vi "Update DropdownMenu.vi"(10 "VacuumLine Obj":refnum<class "VacuumLine.lvclass">, 11 "Controls[]":refnum<vi>[](array[refnum])) -> ()   [LabVIEW 2016, in "Hardware.lvlib" / "VacuumLine.lvlib" / "VacuumLine Configuration.lvclass"]
uses:
  <userlib>/Common Components/Hardware/Abstract System/VacuumLine/VacuumLine Config/VacuumLine Configuration.lvclass
  <userlib>/Common Components/Hardware/Abstract System/VacuumLine/VacuumLine/VacuumLine.lvclass
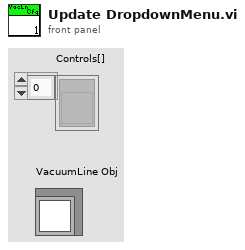
[diagram p1: front panel]
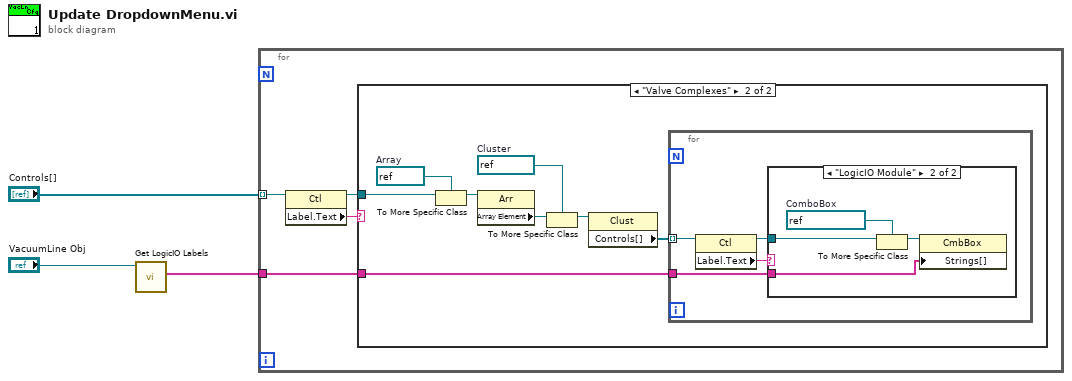
[diagram p0: block diagram]
diagram:
  n1 = call <userlib>:"Get LogicIO Labels.vi"("VacuumLine in"="VacuumLine Obj") -> ("LogicIO Labels"=w2:string[])  [unwired: 8 in, 2 out]
  n2 = for {
    tunnel: "Controls[]" -> [w7] mode=indexing
    tunnel: w2 -> [w4]
    n3 = property class="Ctl"(reference=w7) -> (reference out=w5:refnum<vi>, "Label.Text"=w6:string)  [unwired: 1 in, 1 out]
    n4 = case shown="\"Valve Complexes\"" w6 {
      tunnel: w5 -> [_ w14]
      tunnel: w4 -> [_ w8]
      frame Default {
      }
      frame "Valve Complexes" {
        w12 = refnum<vi> refnum  # Cluster
        w13 = refnum<vi> refnum  # Array
        n5 = To More Specific Class(target class=w13, reference=w14) -> (specific class reference=w15:refnum<vi>)  [unwired: 1 in, 1 out]
        n6 = property class="Arr"(reference=w15) -> ("Array Element"=w11:refnum<vi>)  [unwired: 1 in, 2 out]
        n7 = To More Specific Class(target class=w12, reference=w11) -> (specific class reference=w10:refnum<vi>)  [unwired: 1 in, 1 out]
        n8 = property class="Clust"(reference=w10) -> ("Controls[]"=w9:refnum<vi>[])  [unwired: 1 in, 2 out]
        n9 = for {
          tunnel: w9 -> [w19] mode=indexing
          tunnel: w8 -> [w16]
          n10 = property class="Ctl"(reference=w19) -> (reference out=w17:refnum<vi>, "Label.Text"=w18:string)  [unwired: 1 in, 1 out]
          n11 = case shown="\"LogicIO Module\"" w18 {
            tunnel: w17 -> [_ w22]
            tunnel: w16 -> [_ w20]
            frame Default {
            }
            frame "LogicIO Module" {
              w23 = refnum<vi> refnum  # ComboBox
              n12 = To More Specific Class(target class=w23, reference=w22) -> (specific class reference=w21:refnum<vi>)  [unwired: 1 in, 1 out]
              n13 = property class="CmbBox"(reference=w21, "Strings[]"=w20) -> ()  [unwired: 1 in, 2 out]
            }
          }
        }
      }
    }
  }
